vi "test Custom Device is Disabled.vi"(8 "error in":errorcluster, 11 "TestCase in":refnum<class "Scripting.lvclass">) -> (0 "error out":errorcluster, 3 "TestCase out":refnum<class "Scripting.lvclass">)   [LabVIEW 2020, in "Scripting.lvclass"]
uses:
  Scripting.lvclass
  Scripting/Ballard MIL-STD-1553 Scripting.lvlib
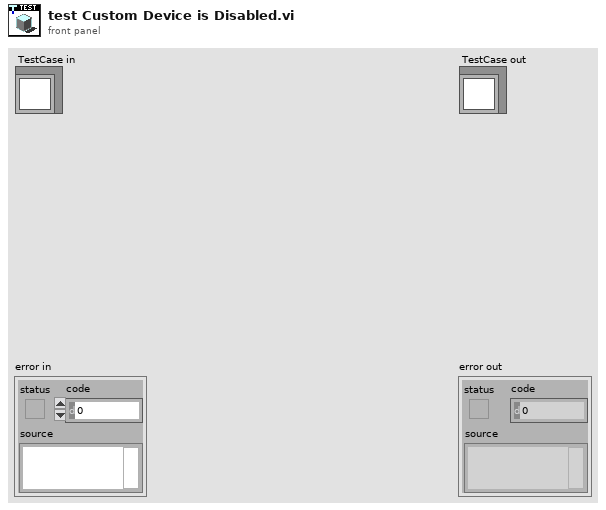
[diagram p1: front panel]
types:
  T1 = typedef "Custom Device API.lvlib/Custom Device Item Ref.ctl" = u64
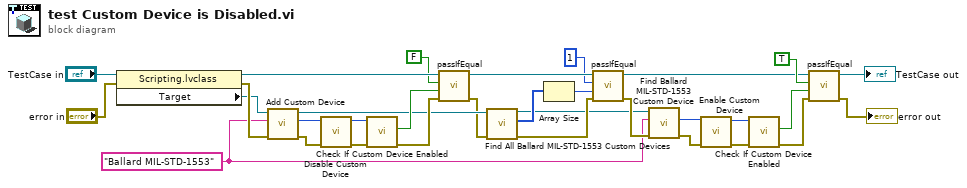
[diagram p0: block diagram]
diagram:
  w3 = "Ballard MIL-STD-1553" ("name")
  n1 = property class="Scripting.lvclass"(reference="TestCase in", error in="error in") -> (reference out=w29:refnum<class "Scripting.lvclass">, error out=w17:errorcluster, "Target"=w14:refnum<k24>)
  n2 = call "Add Custom Device.vi"("error in"=w17, "name"=w3, "target in"=w14) -> ("error out"=w16:errorcluster, "Ballard MIL-STD 1553 custom device"=w15:T1, "target out"=w13:refnum<k24>)  [unwired: 6 in]
  n3 = call "Disable Custom Device.vi"("error in"=w16, "Ballard MIL-STD 1553 custom device in"=w15) -> ("error out"=w30:errorcluster, "Ballard MIL-STD 1553 custom device out"=w31:T1)  [unwired: 8 in]
  n4 = call "Check If Custom Device Enabled.vi"("error in"=w30, "Ballard MIL-STD 1553 custom device in"=w31) -> ("error out"=w26:errorcluster, "Is Custom Device Enabled?"=w27:bool)  [unwired: 7 in, 1 out]
  n5 = call-dynamic "passIfEqual.vi"("error in (no error)"=w26, "y"=w27, "x"=FALSE, "TestCase in"=w29) -> ("error out"=w12:errorcluster, "TestCase out"=w11:refnum<class "Scripting.lvclass">)  [unwired: 6 in]
  n6 = call "Find All Ballard MIL-STD-1553 Custom Devices.vi"("error in"=w12, "target in"=w13) -> ("error out"=w9:errorcluster, "Ballard MIL-STD-1553 custom devices"=w8:T1[], "target out"=w4:refnum<k24>)  [unwired: 7 in]
  n7 = Array Size(array=w8) -> (size(s)=w7:i32)
  n8 = call-dynamic "passIfEqual.vi"("error in (no error)"=w9, "y"=w7, "x"=1, "TestCase in"=w11) -> ("error out"=w5:errorcluster, "TestCase out"=w10:refnum<class "Scripting.lvclass">)  [unwired: 6 in]
  n9 = call "Find Ballard MIL-STD-1553 Custom Device.vi"("error in"=w5, "name"=w3, "target in"=w4) -> ("error out"=w1:errorcluster, "Ballard MIL-STD 1553 custom device"=w2:T1)  [unwired: 5 in, 2 out]
  n10 = call "Enable Custom Device.vi"("error in"=w1, "Ballard MIL-STD 1553 custom device in"=w2) -> ("error out"=w24:errorcluster, "Ballard MIL-STD 1553 custom device out"=w25:T1)  [unwired: 8 in]
  n11 = call "Check If Custom Device Enabled.vi"("error in"=w24, "Ballard MIL-STD 1553 custom device in"=w25) -> ("error out"=w22:errorcluster, "Is Custom Device Enabled?"=w21:bool)  [unwired: 7 in, 1 out]
  n12 = call-dynamic "passIfEqual.vi"("error in (no error)"=w22, "y"=w21, "x"=TRUE, "TestCase in"=w10) -> ("error out"=→"error out":errorcluster, "TestCase out"=→"TestCase out":refnum<class "Scripting.lvclass">)  [unwired: 6 in]
